vi "Get CVT Data.vi"(7 "Subgroup":string, 8 "error in":errorcluster, 9 "Variable":string, 10 "Group":string, 11 "CVT Session In":T1) -> (0 "error out":errorcluster, 1 "found":bool, 2 "Data Out":variant, 3 "CVT Session Out":T1)   [LabVIEW 2015, in "CVT.lvclass"]
uses:
  CVT.lvclass
  <vilib>/MSR Consulting, LLC/General Reuse/Session APIs/_Session Fwk/Typedefs/Session Handle.ctl
  <vilib>/MSR Consulting, LLC/General Reuse/Session APIs/_Session Fwk/Session - Root.lvclass
  CVT.lvclass/CVT.ctl
  Read CVT.vi
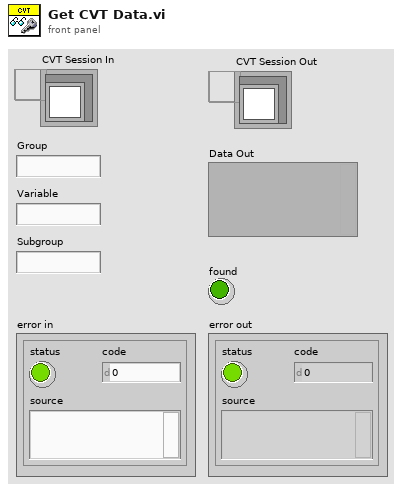
[diagram p1: front panel]
types:
  T1 = typedef "Session - Root.lvclass/Session Handle.ctl" = refnum<data-value>
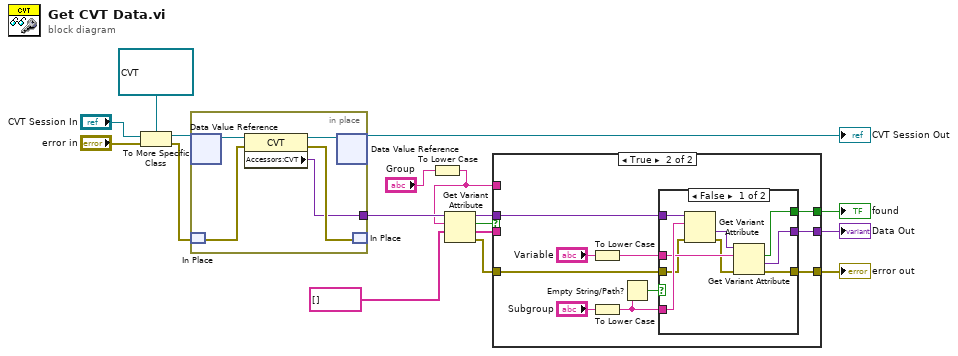
[diagram p0: block diagram]
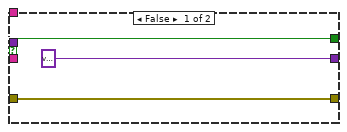
[diagram p2: hidden frame]
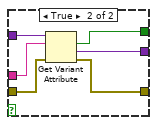
[diagram p3: hidden frame]
diagram:
  n1 = To More Specific Class(target class=refnum<data-value> refnum ("CVT Session In"), reference="CVT Session In", error in="error in") -> (specific class reference=w15:refnum<data-value>, error out=w14:errorcluster)
  n2 = in-place {
    in-place-border: [w18] -> w11
    n3 = in-place-dvr #1(w15) -> (w22:refnum<class "CVT.lvclass">)  [unwired: 1 out]
    n4 = in-place-match #2(w14) -> (w21:errorcluster)
    n5 = property class="CVT"(reference=w22, error in=w21) -> (reference out=w20:refnum<class "CVT.lvclass">, error out=w19:errorcluster, "Accessors:CVT"=w18:variant)
    n6 = in-place-dvr #1(w20) -> (→"CVT Session Out":refnum<data-value>)  [unwired: 1 out]
    n7 = in-place-match #2(w19) -> ()  [unwired: 1 out]
  }
  n8 = To Lower Case(string="Group") -> (all lower case string=w1:string)
  n9 = Get Variant Attribute(Variant=w11, name=w1, default value (empty Variant)=string[] []) -> (duplicate Variant=w9:variant, found=w8:bool, value=w3:string[], error out=w7:errorcluster)  [unwired: 1 in]
  n10 = case shown="True" w8 {
    selector: w8 -> [w24 _]
    tunnel: w9 -> [_ w35]
    tunnel: w7 -> [w25 w30]
    tunnel: w1 -> [_ _]
    tunnel: [variant w33] -> w6
    tunnel: [w24 w32] -> w5
    tunnel: [w25 w31] -> w4
    tunnel: w3 -> [_ _]
    frame False {
    }
    frame True {
      n11 = To Lower Case(string="Variable") -> (all lower case string=w28:string)
      n12 = To Lower Case(string="Subgroup") -> (all lower case string=w26:string)
      n13 = Empty String/Path?(string/path=w26) -> (empty?=w34:bool)
      n14 = case shown="False" w34 {
        tunnel: w35 -> [w44 w50]
        tunnel: w28 -> [w41 w49]
        tunnel: [w40 w48] -> w33
        tunnel: [w39 w47] -> w32
        tunnel: w26 -> [w43 _]
        tunnel: [w37 w46] -> w31
        tunnel: w30 -> [w36 w45]
        frame False {
          n15 = Get Variant Attribute(Variant=w44, name=w43, error in=w36) -> (value=w42:variant, error out=w38:errorcluster)  [unwired: 1 in, 2 out]
          n16 = Get Variant Attribute(Variant=w42, name=w41, error in=w38) -> (found=w39:bool, value=w40:variant, error out=w37:errorcluster)  [unwired: 1 in, 1 out]
        }
        frame True {
          n17 = Get Variant Attribute(Variant=w50, name=w49, error in=w45) -> (found=w47:bool, value=w48:variant, error out=w46:errorcluster)  [unwired: 1 in, 1 out]
        }
      }
    }
  }
  "found" <- w5
  "error out" <- w4
  "Data Out" <- w6
